vi "S2C_FORNAX_Proc_Initialize.vi"(8 "Error In":errorcluster) -> (0 "Error Out":errorcluster)   [LabVIEW 2015]
uses:
  _Shared/S2C_Shared_Proc_Globals.vi
  S2C_FORNAX_Proc_Globals.vi
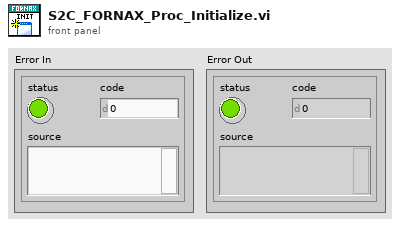
[diagram p1: front panel]
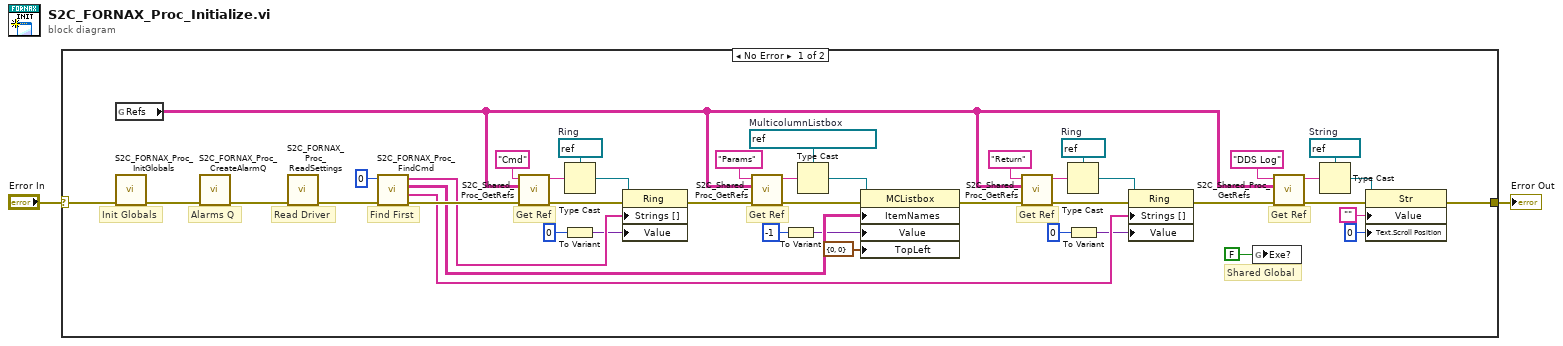
[diagram p0: block diagram]
diagram:
  n1 = case shown="No Error" "Error In" {
    selector: "Error In" -> [w5 w47]
    tunnel: [w8 w47] -> w1
    frame No Error {
      w14 = refnum<vi> refnum  # String
      w28 = refnum<vi> refnum  # Ring
      w36 = refnum<vi> refnum  # MulticolumnListbox
      w42 = refnum<vi> refnum  # Ring
      # "Alarms Q"
      # "Init Globals"
      # "Shared Global"
      # "Get Ref"
      # "Get Ref"
      # "Get Ref"
      # "Get Ref"
      # "Find First"
      # "Read Driver"
      n2 = global read "S2C_FORNAX_Proc_Globals.vi" "Refs"() -> (w6:string[][])
      n3 = call "S2C_FORNAX_Proc_InitGlobals.vi"("Error In"=w5) -> ("Error Out"=w4:errorcluster)  [unwired: 10 in]
      n4 = call "S2C_FORNAX_Proc_CreateAlarmQ.vi"("Error In"=w4) -> ("Error Out"=w3:errorcluster)  [unwired: 10 in]
      n5 = call "S2C_FORNAX_Proc_ReadSettings.vi"("Error In"=w3) -> ("Error Out"=w46:errorcluster)  [unwired: 10 in]
      n6 = call "S2C_FORNAX_Proc_FindCmd.vi"("Error In"=w46, "Index"=0) -> ("Error Out"=w39:errorcluster, "Returns"=w24:string[], "Parameters"=w31:string[][], "AllCmds"=w32:string[])  [unwired: 6 in]
      n7 = call "S2C_Shared_Proc_GetRefs.vi"("Error In"=w39, "Refs"=w6, "Label"="Cmd") -> ("Error Out"=w41:errorcluster, "Reference"=w43:string)  [unwired: 7 in]
      n8 = Type Cast(type=w42, x=w43) -> (*(type *) &x=w44:refnum<vi>)
      n9 = To Variant(anything=0) -> (Variant=w22:variant)
      n10 = property class="Ring"(reference=w44, error in=w41, "Strings []"=w32, "Value"=w22) -> (error out=w33:errorcluster)  [unwired: 1 out]
      n11 = call "S2C_Shared_Proc_GetRefs.vi"("Error In"=w33, "Refs"=w6, "Label"="Params") -> ("Error Out"=w37:errorcluster, "Reference"=w35:string)  [unwired: 7 in]
      n12 = To Variant(anything=-1) -> (Variant=w17:variant)
      n13 = Type Cast(type=w36, x=w35) -> (*(type *) &x=w34:refnum<vi>)
      n14 = property class="MCListbox"(reference=w34, error in=w37, "ItemNames"=w31, "Value"=w17, "TopLeft"=cluster{"Row":u32, "Column":u32} {"Row"=0, "Column"=0} ("Top Left Visible Cell")) -> (error out=w25:errorcluster)  [unwired: 1 out]
      n15 = call "S2C_Shared_Proc_GetRefs.vi"("Error In"=w25, "Refs"=w6, "Label"="Return") -> ("Error Out"=w29:errorcluster, "Reference"=w27:string)  [unwired: 7 in]
      n16 = Type Cast(type=w28, x=w27) -> (*(type *) &x=w26:refnum<vi>)
      n17 = To Variant(anything=0) -> (Variant=w19:variant)
      n18 = property class="Ring"(reference=w26, error in=w29, "Strings []"=w24, "Value"=w19) -> (error out=w11:errorcluster)  [unwired: 1 out]
      n19 = global write "S2C_Shared_Proc_Globals.vi" "Exe?"(FALSE ("Exe?")) -> ()
      n20 = call "S2C_Shared_Proc_GetRefs.vi"("Error In"=w11, "Refs"=w6, "Label"="DDS Log") -> ("Error Out"=w13:errorcluster, "Reference"=w15:string)  [unwired: 7 in]
      n21 = Type Cast(type=w14, x=w15) -> (*(type *) &x=w16:refnum<vi>)
      n22 = property class="Str"(reference=w16, error in=w13, "Value"="", "Text.Scroll Position"=u32 0) -> (error out=w8:errorcluster)  [unwired: 1 out]
    }
    frame Error {
    }
  }
  "Error Out" <- w1
